vi "rename_lib2.vi"(10 "Variant":variant) -> (0 "error out":errorcluster)   [LabVIEW 2019]
panel:
  # "THIS IS A PLACEHOLDER VI\nIt was created accidentally by a VIPM bug corrected in 2012.1\nHowever, the option calling this VI cannot be removed\nDo not include in built package"
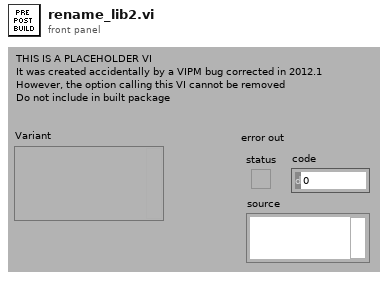
[diagram p1: front panel]
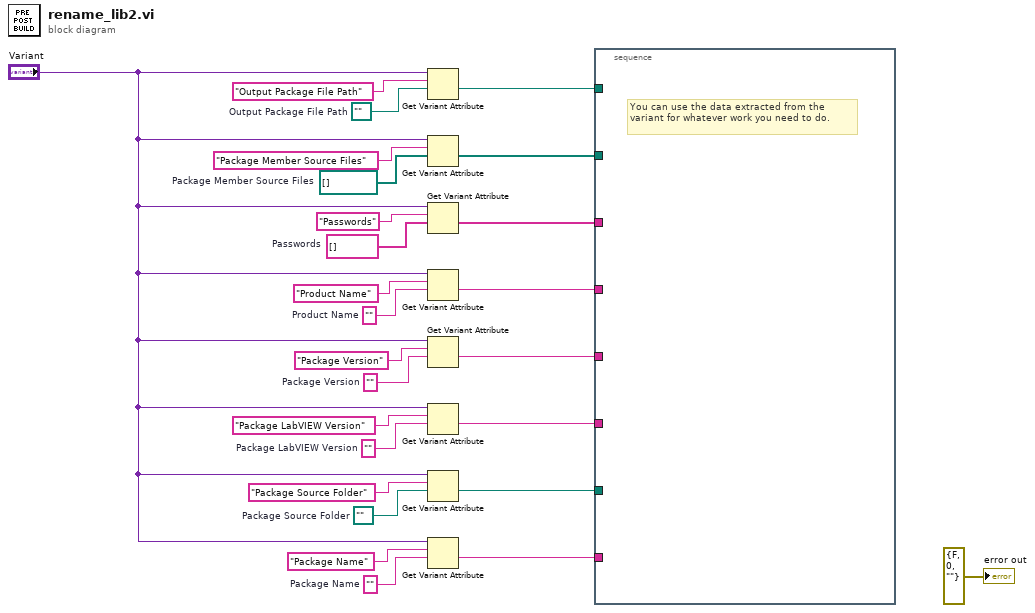
[diagram p0: block diagram]
diagram:
  w9 = path ""  # Package Source Folder
  w10 = ""  # Package Name
  w13 = ""  # Package LabVIEW Version
  w15 = ""  # Package Version
  w17 = ""  # Product Name
  w21 = string[] []  # Passwords
  w23 = path[] []  # Package Member Source Files
  w25 = path ""  # Output Package File Path
  n1 = Get Variant Attribute(Variant="Variant", name="Output Package File Path", default value (empty Variant)=w25) -> (value=w8:path)  [unwired: 1 in, 3 out]
  n2 = Get Variant Attribute(Variant="Variant", name="Package Member Source Files", default value (empty Variant)=w23) -> (value=w7:path[])  [unwired: 1 in, 3 out]
  n3 = Get Variant Attribute(Variant="Variant", name="Passwords", default value (empty Variant)=w21) -> (value=w6:string[])  [unwired: 1 in, 3 out]
  n4 = Get Variant Attribute(Variant="Variant", name="Product Name", default value (empty Variant)=w17) -> (value=w5:string)  [unwired: 1 in, 3 out]
  n5 = Get Variant Attribute(Variant="Variant", name="Package Version", default value (empty Variant)=w15) -> (value=w4:string)  [unwired: 1 in, 3 out]
  n6 = Get Variant Attribute(Variant="Variant", name="Package LabVIEW Version", default value (empty Variant)=w13) -> (value=w3:string)  [unwired: 1 in, 3 out]
  n7 = Get Variant Attribute(Variant="Variant", name="Package Source Folder", default value (empty Variant)=w9) -> (value=w2:path)  [unwired: 1 in, 3 out]
  n8 = Get Variant Attribute(Variant="Variant", name="Package Name", default value (empty Variant)=w10) -> (value=w1:string)  [unwired: 1 in, 3 out]
  n9 = stacked-sequence {
    tunnel: w8 -> [_]
    tunnel: w7 -> [_]
    tunnel: w6 -> [_]
    tunnel: w5 -> [_]
    tunnel: w4 -> [_]
    tunnel: w3 -> [_]
    tunnel: w2 -> [_]
    tunnel: w1 -> [_]
    frame #0 {
      # "You can use the data extracted from the variant for whatever work you need to do."
    }
  }
  "error out" <- errorcluster {"status"=FALSE, "code"=0, "source"=""} ("error out")
